vi "Actor Loop.vi"(11 "Actor in":refnum<class "Actor.lvclass">) -> ()   [LabVIEW 2021, in "jettl.lvlib" / "Actor.lvclass"]
uses:
  Actor.lvclass
  Msg Strategy/Msg Strategy.lvclass
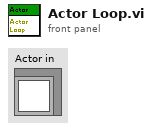
[diagram p1: front panel]
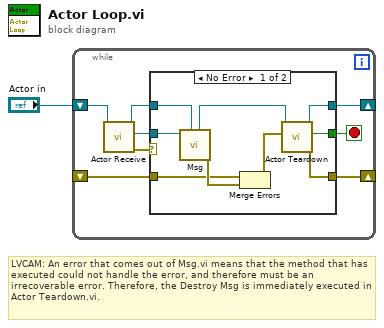
[diagram p0: block diagram]
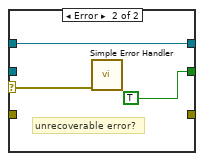
[diagram p2: hidden frame]
diagram:
  # "LVCAM: An error that comes out of Msg.vi means that the method that has executed could not handle the error, and therefore must be an irrecoverable error. Therefore, the Destroy Msg is immediately executed in Actor Teardown.vi."
  n1 = while {
    shift-right: [w9] -> _
    shift-left: "Actor in" -> [w3]
    shift-right: [w5] -> _
    shift-left: _ -> [w4]
    stop <- w7 stop-if-true
    n2 = call-dynamic "Actor Receive.vi"("Actor in"=w3) -> ("error out"=w6:errorcluster, "Msg"=w8:refnum<class "Msg Strategy.lvclass">, "Actor out"=w2:refnum<class "Actor.lvclass">)  [unwired: 8 in]
    n3 = case shown="No Error" w6 {
      selector: w6 -> [_ w19]
      tunnel: [w10 w21] -> w9
      tunnel: w8 -> [w18 _]
      tunnel: [w16 TRUE ("Destroyed Self?")] -> w7
      tunnel: w2 -> [w17 w21]
      tunnel: [w15 _] -> w5
      tunnel: w4 -> [w12 _]
      frame No Error {
        n4 = call-dynamic "Msg.vi"("Actor in"=w17, "Msg Strategy in"=w18) -> ("error out"=w13:errorcluster, "Actor out"=w11:refnum<class "Actor.lvclass">)  [unwired: 8 in]
        n5 = Merge Errors(w12, w13) -> (w14:errorcluster)
        n6 = call-dynamic "Actor Teardown.vi"("Error"=w14, "Actor in"=w11) -> ("error out"=w15:errorcluster, "Teardown?"=w16:bool, "Actor out"=w10:refnum<class "Actor.lvclass">)  [unwired: 7 in]
      }
      frame Error {
        # "unrecoverable error?"
        n7 = call <vilib>:"Simple Error Handler.vi"("error in (no error)"=w19) -> ()  [unwired: 4 in, 5 out]
      }
    }
  }
